vi "Send Data for UI.vi"(0 "Measure Call Context in":refnum<class "Measure Call Context.lvclass">, 1 "fpga interface in":refnum<k20>, 3 "Last displayed image data":u32[](array[numeric]), 5 "FrameCount":u64, 9 "References":T1, 11 "error in":errorcluster, 12 "Status data":T3, 13 "SOURCE RATE (fps)":dbl, 14 "Active Channel":string) -> (15 "error out":errorcluster)   [LabVIEW 2025, in "Automotive Vision.lvclass"]
doc: "Handles data transfer to the UI."
uses:
  Automotive Vision.lvclass
  Automotive Vision.lvclass/Automotive Vision.ctl
  Measurement Results.ctl
  <vilib>/Plug-In SDKs/Measurements/Measure Call Context/Measure Call Context.lvclass
  <instrlib>/FlexRIO/CSI-2/v2/Common/Types/LLP Data Type.ctl
  <instrlib>/FlexRIO/CSI-2/v2/Common/NI CSI-2 API Common v2.lvlib
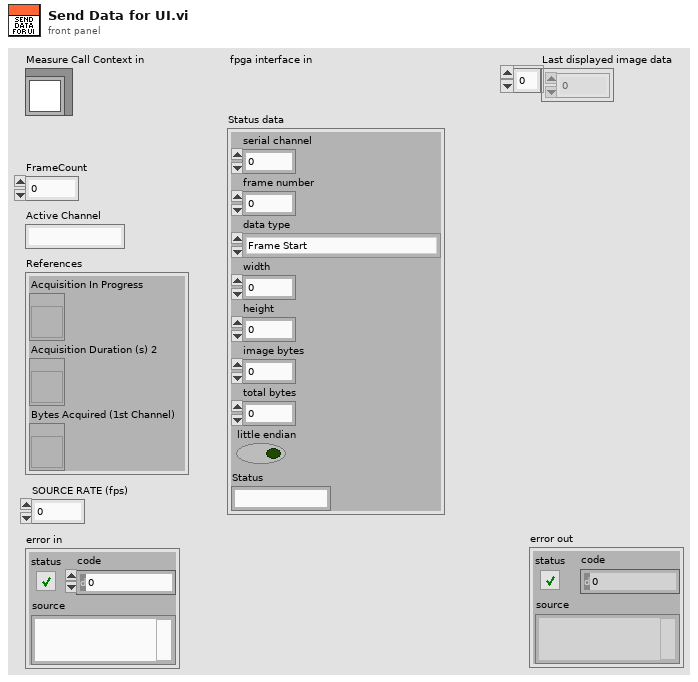
[diagram p1: front panel]
types:
  T1 = cluster{"Acquisition In Progress":refnum<vi>, "Acquisition Duration (s) 2":refnum<vi>, "Bytes Acquired (1st Channel)":refnum<vi>}
  T2 = typedef "NI CSI-2 API Common v2.lvlib/LLP Data Type.ctl" = enum8{"Frame Start", "Frame End", "Line Start", "Line End", "End of Transmission", "Reserved 0", "Reserved 1", "Reserved 2", "Generic Short Packet 1", "Generic Short Packet 2", "Generic Short Packet 3", "Generic Short Packet 4", "Generic Short Packet 5", "Generic Short Packet 6", "Generic Short Packet 7", "Generic Short Packet 8", "Null", "Blanking Data", "Embedded 8-bit non Image Data", "Generic Long Packet 1", "Generic Long Packet 2", "Generic Long Packet 3", "Generic Long Packet 4", "Reserved 3", "YUV420 8-bit", "YUV420 10-bit", "Legacy YUV420 8-bit", "Reserved 4", "YUV420 8-bit Chroma Shifted", "YUV420 10-bit Chroma Shifted", "YUV422 8-bit", "YUV422 10-bit", "RGB444", "RGB555", "RGB565", "RGB666", "RGB888", "Reserved 5", "Reserved 6", "RAW 24", "RAW 6", "RAW 7", "RAW 8", "RAW 10", "RAW 12", "RAW 14", "RAW 16", "RAW 20", "User Defined 8-bit Data 1", "User Defined 8-bit Data 2", "User Defined 8-bit Data 3", "User Defined 8-bit Data 4", "User Defined 8-bit Data 5", "User Defined 8-bit Data 6", "User Defined 8-bit Data 7", "User Defined 8-bit Data 8", "USL Command", "Reserved 7", "Reserved 8", "Reserved 9", "Reserved 10", "Reserved 11", "Reserved 12", "LRTE EPD Spacer"}
  T3 = cluster{"serial channel":fxp<+,3,3>, "frame number":u16, "data type":T2, "width":u16, "height":u16, "image bytes":u32, "total bytes":u32, "little endian":bool, "Status":string}
  T4 = typedef "Automotive Vision.lvclass/Measurement Results.ctl" = cluster{"ACQ. IN PROGRESS":bool, "IMAGE PIXEL DATA":u32[], "ACQ. DURATION (s)":dbl, "SOURCE RATE (fps)":dbl, "BYTES ACQUIRED":u64, "FRAME COUNT":u64, "POC VOLTAGE (V)":dbl, "POC CURRENT (A)":dbl, "ERROR":bool, "STATE MESSAGE":string, "IMAGE DATA":string, "OOB gRPC Port":i32, "HEIGHT":u64, "WIDTH":u64}
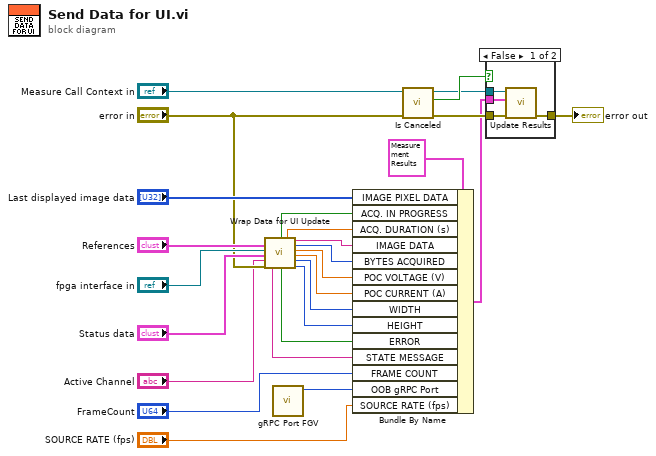
[diagram p0: block diagram]
diagram:
  n1 = call "Wrap Data for UI Update.vi"("References"="References", "fpga inteface in"="fpga interface in", "image metadata"="Status data", "Active Channel"="Active Channel", "error in"="error in") -> ("State message"=w14:string, "Acqusition In Progress"=w9:bool, "status"=w13:bool, "Acquisition Duration"=w10:dbl, "Image Data"=w4:string, "Bytes Acquired"=w5:u64, "PowerOverCoaxCurrent"=w11:dbl, "PowerOverCoaxVoltage"=w12:dbl, "width"=w24:u64, "height"=w25:u64)  [unwired: 5 in]
  n2 = call "gRPC Port FGV.vi"() -> ("Listening Port out"=w23:i32)  [unwired: 11 in]
  n3 = Bundle By Name(cluster=T4 {"ACQ. IN PROGRESS"=FALSE, "IMAGE PIXEL DATA"=[], "ACQ. DURATION (s)"=0.0, "SOURCE RATE (fps)"=0.0, "BYTES ACQUIRED"=0, "FRAME COUNT"=0, "POC VOLTAGE (V)"=0.0, "POC CURRENT (A)"=0.0, "ERROR"=FALSE, "STATE MESSAGE"="", "IMAGE DATA"="", "OOB gRPC Port"=0, "HEIGHT"=0, "WIDTH"=0} ("Measurement Results"), "IMAGE PIXEL DATA"="Last displayed image data", "ACQ. IN PROGRESS"=w9, "ACQ. DURATION (s)"=w10, "IMAGE DATA"=w4, "BYTES ACQUIRED"=w5, "POC VOLTAGE (V)"=w11, "POC CURRENT (A)"=w12, "WIDTH"=w24, "HEIGHT"=w25, "ERROR"=w13, "STATE MESSAGE"=w14, "FRAME COUNT"="FrameCount", "OOB gRPC Port"=w23, "SOURCE RATE (fps)"="SOURCE RATE (fps)") -> (w7:T4)
  n4 = call <vilib>:"Is Canceled.vi"("error in"="error in", "measure call context in"="Measure Call Context in") -> ("error out"=w22:errorcluster, "is canceled?"=w21:bool, "measure call context out"=w20:refnum<class "Measure Call Context.lvclass">)  [unwired: 7 in]
  n5 = case shown="False" w21 {
    tunnel: w7 -> [w30 _]
    tunnel: [w29 w31] -> w8
    tunnel: w20 -> [w28 _]
    tunnel: w22 -> [w27 w31]
    frame False {
      n6 = call <vilib>:"Update Results.vi"("error in"=w27, "measurement results"=w30, "measure call context in"=w28) -> ("error out"=w29:errorcluster)  [unwired: 7 in, 1 out]
    }
    frame True {
    }
  }
  "error out" <- w8
